vi "NextField.vi"(0 "const phi?":bool, 5 "sweep parameter":T1=enum."magnetic field", 7 "target mag (T)":dbl[](array[numeric]), 9 "phi array (deg)":dbl[](array[numeric]), 12 "Loop index":i32) -> (8 "Next mag (T)":dbl format="%#_13g", 10 "Next phi (deg)":dbl format="%#_13g", 13 "Loop Count":i32)   [LabVIEW 2013]
uses:
  measurement/measurement sweep parameter.ctl
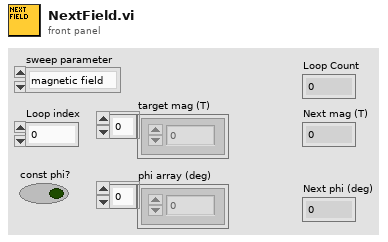
[diagram p1: front panel]
types:
  T1 = typedef "measurement sweep parameter.ctl" = enum16{"angle", "magnetic field"}
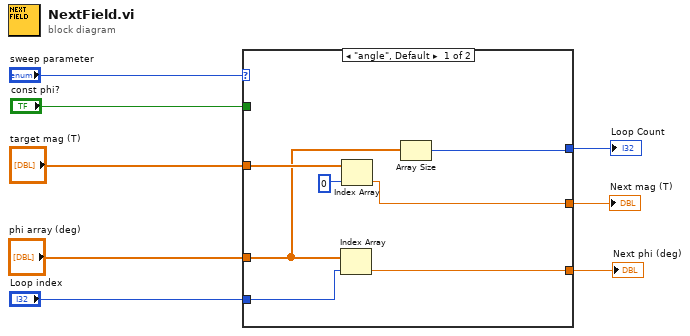
[diagram p0: block diagram]
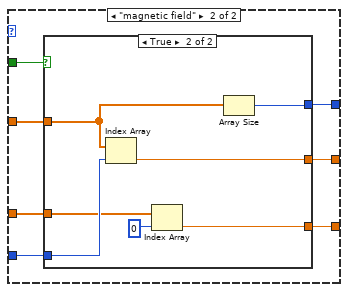
[diagram p2: hidden frame]
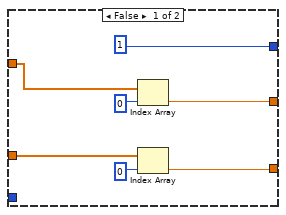
[diagram p3: hidden frame]
diagram:
  n1 = case shown="\"angle\", Default" "sweep parameter" {
    tunnel: "target mag (T)" -> [w12 w22]
    tunnel: "Loop index" -> [w15 w21]
    tunnel: [w11 w20] -> w6
    tunnel: "phi array (deg)" -> [w9 w18]
    tunnel: [w14 w19] -> w4
    tunnel: "const phi?" -> [_ w17]
    tunnel: [w10 w16] -> w1
    frame "angle", Default {
      n2 = Index Array(array=w9, index=w15) -> (element=w14:dbl)
      n3 = Index Array(array=w12, index=0 ("Loop index 2")) -> (element=w11:dbl)
      n4 = Array Size(array=w9) -> (size(s)=w10:i32)
    }
    frame "magnetic field" {
      n5 = case shown="True" w17 {
        tunnel: w22 -> [w27 w30]
        tunnel: w21 -> [_ w36]
        tunnel: [w28 w35] -> w20
        tunnel: [w24 w33] -> w19
        tunnel: w18 -> [w25 w32]
        tunnel: [1 ("Loop index 2") w31] -> w16
        frame False {
          n6 = Index Array(array=w27, index=0 ("Loop index 2")) -> (element=w28:dbl)
          n7 = Index Array(array=w25, index=0 ("Loop index 2")) -> (element=w24:dbl)
        }
        frame True {
          n8 = Index Array(array=w30, index=w36) -> (element=w35:dbl)
          n9 = Index Array(array=w32, index=0 ("Loop index 2")) -> (element=w33:dbl)
          n10 = Array Size(array=w30) -> (size(s)=w31:i32)
        }
      }
    }
  }
  "Next mag (T)" <- w6
  "Next phi (deg)" <- w4
  "Loop Count" <- w1
